vi "Temperature Monitor.vi"() -> ()   [LabVIEW 2017]
doc: "This VI is the solution to an exercise in the LabVIEW Core 1 course.\n\nIt uses a While Loop and shift registers to average data. No hardware is necessary."
panel:
  in  "Stop Button":bool
  out "Temperature History":cluster{dbl, "Temperature Value":dbl}(graph)
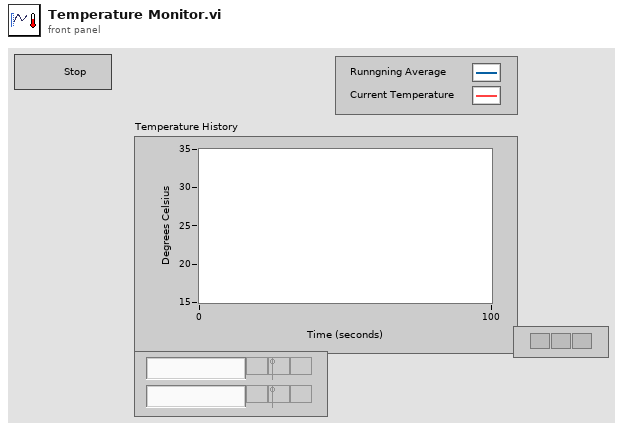
[diagram p1: front panel]
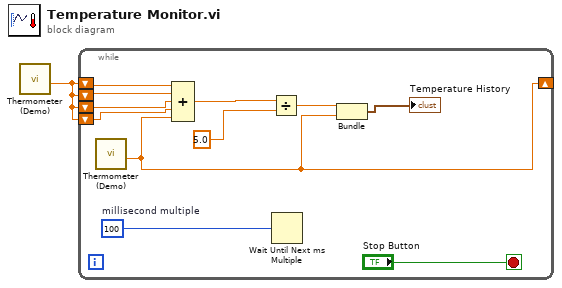
[diagram p0: block diagram]
diagram:
  n1 = call "Thermometer (Demo).vi"() -> ("Temperature Value"=w1:dbl)  [unwired: 11 in]
  n2 = while {
    shift-right: [w3] -> _
    shift-left: w1 -> [w7]
    shift-left: w1 -> [w6]
    shift-left: w1 -> [w5]
    shift-left: w1 -> [w8]
    stop <- "Stop Button" stop-if-true
    w12 = u32 100  # millisecond multiple
    n3 = call "Thermometer (Demo).vi"() -> ("Temperature Value"=w3:dbl)  [unwired: 11 in]
    n4 = Compound Arithmetic op=ADD(w8, w7, w6, w5, w3) -> (w10:dbl)
    n5 = Divide(x=w10, y=5.0) -> (x/y=w4:dbl)
    n6 = Wait Until Next ms Multiple(millisecond multiple=w12) -> ()  [unwired: 1 out]
    n7 = Bundle(w4, "Temperature Value"=w3) -> (→"Temperature History":cluster{dbl, "Temperature Value":dbl})  [unwired: 1 in]
  }
